vi "Gyro PID Fwd Dis.vi"(6 "Target angle":sgl, 7 "Threshold to stop":i32=1200, 8 "Threshold to slow":i32=1000, 9 "Min. speed":i32=40, 10 "Max. speed":i32=80, 11 "EV3 in":T1) -> (3 "EV3 out":T1)   [LabVIEW 2016]
uses:
  <vilib>/NXT/Subs/LVHSConnector.ctl
  <vilib>/NXT/LegoClasses/BrickReference/BrickReference.lvclass
  <vilib>/NXT/Block Support/NXT_OutputPort.ctl
  <vilib>/NXT/NXTIO Xnodes/NXTIONodeSubVIs/LEGOResetMotors.vi
  <vilib>/NXT/Dual Mode Library/Motors/Rotation.vi
  <vilib>/NXT/NXTIO Xnodes/NXTIONodeSubVIs/NXTMotorSteeringOn.vi
  <vilib>/NXT/NXTIO Xnodes/NXTIONodeSubVIs/NXTStopMotors.vi
  <vilib>/NXT/Dual Mode Library/Waits/Wait_Num.vi
  <vilib>/NXT/NXTIO Xnodes/NXTIOXNode/NXTIO.xnode
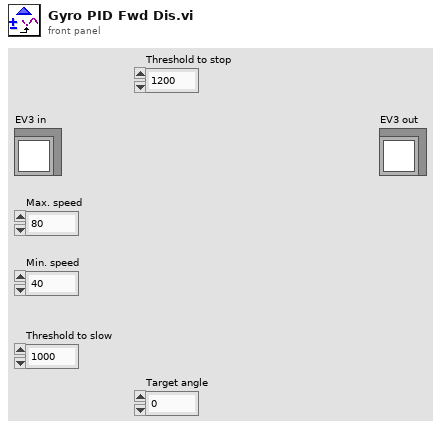
[diagram p1: front panel]
types:
  T1 = typedef "LVHSConnector.ctl" = refnum<class "BrickReference.lvclass">
  T2 = typedef "NXT_OutputPort.ctl" = u8
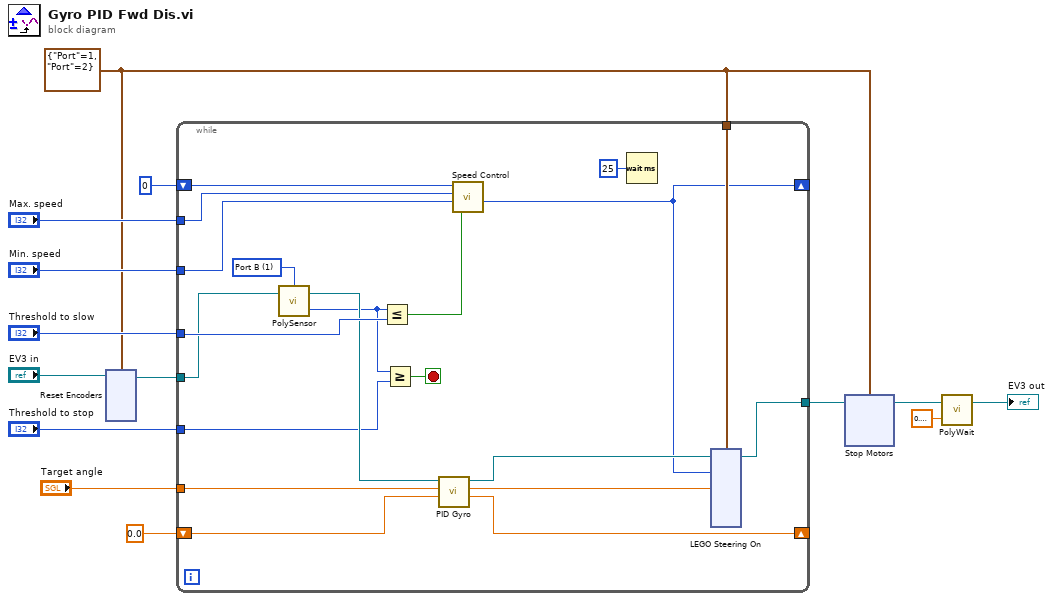
[diagram p0: block diagram]
diagram:
  w4 = cluster{"Port":T2, "Port":T2} {"Port"=1, "Port"=2} ("Motor")
  n1 = xnode "Reset Encoders"("Motors"=w4, "NXT/EV3"="EV3 in") -> ("NXT/EV3"=w10:T1)
  n2 = while {
    tunnel: w10 -> [w23]
    shift-right: [w34] -> _
    shift-left: sgl 0.0 -> [w17]
    tunnel: "Target angle" -> [w33]
    tunnel: [w30] -> w6
    tunnel: w4 -> [w32]
    shift-right: [w16] -> _
    shift-left: 0 -> [w27]
    tunnel: "Min. speed" -> [w24]
    tunnel: "Max. speed" -> [w26]
    tunnel: "Threshold to slow" -> [w25]
    tunnel: "Threshold to stop" -> [w15]
    stop <- w20 stop-if-true
    w31 = T2 1 items=["Port A", "Port B", "Port C", "Port D"] ("Port (Port A)")
    n3 = call-poly <vilib>:"PolySensor.vi"("NXT/EV3"=w23, "Port (Port A)"=w31) -> ("Angle of Rotation"=w19:i32, "NXT/EV3"=w22:T1)  [unwired: 1 in]
    n4 = Less Or Equal?(x=w19, y=w25) -> (x <= y?=w21:bool)
    n5 = Greater Or Equal?(x=w19, y=w15) -> (x >= y?=w20:bool)
    n6 = call "PID Gyro.vi"("Previous integral"=w17, "Target angle"=w33, "EV3 in"=w22) -> ("New integral"=w34:sgl, "Total error"=w28:sgl, "EV3 out"=w18:T1)  [unwired: 6 in]
    n7 = call "Speed Control.vi"("Speed Up or Down?"=w21, "Min. speed"=w24, "Max. speed"=w26, "Ini. speed"=w27) -> ("Speed out"=w16:i32)  [unwired: 7 in]
    n8 = Wait (ms)(milliseconds to wait=u32 25) -> ()  [unwired: 1 out]
    n9 = xnode "LEGO Steering On"("Steering 1"=w28, "Power 1"=w16, "Motors"=w32, "NXT/EV3"=w18) -> ("NXT/EV3"=w30:T1)
  }
  n10 = xnode "Stop Motors"("Motors"=w4, "NXT/EV3"=w6) -> ("NXT/EV3"=w5:T1)
  n11 = call-poly <vilib>:"PolyWait.vi"("Time (1 sec)"=sgl 0.2, "NXT/EV3"=w5) -> ("NXT/EV3"=→"EV3 out":T1)  [unwired: 2 in]
